vi "read_IMU_two_datasets_scaled.vi"(0 "First Measurement Type":u16(ring)=4608 items=["PAGE-ID"=0, "SYS_E_FLAG"=2048, "DIAG_STS"=2560, "ALM_STS"=3072, "TEMP_OUT"=3584, "X_GYRO_OUT"=4608, "Y_GYRO_OUT"=5632, "Z_GYRO_OUT"=6656, "X_ACCL_OUT"=7680, "Y_ACCL_OUT"=8704, "Z_ACCL_OUT"=9728, "X_MAGN_OUT"=10240, "Y_MAGN_OUT"=10752, "Z_MAGN_OUT"=11264, "BAROM_OUT"=12288, "X_DELTAANG_OUT"=16896, "Y_DELTAANG_OUT"=17920, "Z_DELTAANG_OUT"=18944, "X_DELTAVEL_OUT"=19968, "Y_DELTAVEL_OUT"=20992, "Z_DELTAVEL_OUT"=22016], 3 "Last Measurement Type":u16(ring)=4608 items=["PAGE-ID"=0, "SYS_E_FLAG"=2048, "DIAG_STS"=2560, "ALM_STS"=3072, "TEMP_OUT"=3584, "X_GYRO_OUT"=4608, "Y_GYRO_OUT"=5632, "Z_GYRO_OUT"=6656, "X_ACCL_OUT"=7680, "Y_ACCL_OUT"=8704, "Z_ACCL_OUT"=9728, "X_MAGN_OUT"=10240, "Y_MAGN_OUT"=10752, "Z_MAGN_OUT"=11264, "BAROM_OUT"=12288, "X_DELTAANG_OUT"=16896, "Y_DELTAANG_OUT"=17920, "Z_DELTAANG_OUT"=18944, "X_DELTAVEL_OUT"=19968, "Y_DELTAVEL_OUT"=20992, "Z_DELTAVEL_OUT"=22016], 7 "Gravitation-Constant":dbl=9.81, 9 "Next Measurement Type":u16(ring)=4608 items=["PAGE-ID"=0, "SYS_E_FLAG"=2048, "DIAG_STS"=2560, "ALM_STS"=3072, "TEMP_OUT"=3584, "X_GYRO_OUT"=4608, "Y_GYRO_OUT"=5632, "Z_GYRO_OUT"=6656, "X_ACCL_OUT"=7680, "Y_ACCL_OUT"=8704, "Z_ACCL_OUT"=9728, "X_MAGN_OUT"=10240, "Y_MAGN_OUT"=10752, "Z_MAGN_OUT"=11264, "BAROM_OUT"=12288, "X_DELTAANG_OUT"=16896, "Y_DELTAANG_OUT"=17920, "Z_DELTAANG_OUT"=18944, "X_DELTAVEL_OUT"=19968, "Y_DELTAVEL_OUT"=20992, "Z_DELTAVEL_OUT"=22016], 11 "error in (no error)":errorcluster) -> (1 "Sensor 1":string, 5 "Unit  1":string, 6 "Scaled Measurement 1":dbl, 10 "Scaled last Measurement":dbl, 12 "Last Sensor":string, 14 "error out":errorcluster, 15 "Last Unit":string)   [LabVIEW 2013]
panel:
  out "Error array 2":bool[](array[boolean])
  out "Error  array 1":bool[](array[boolean])
  out "1st Dataset":i16
  out "Last Dataset":i16
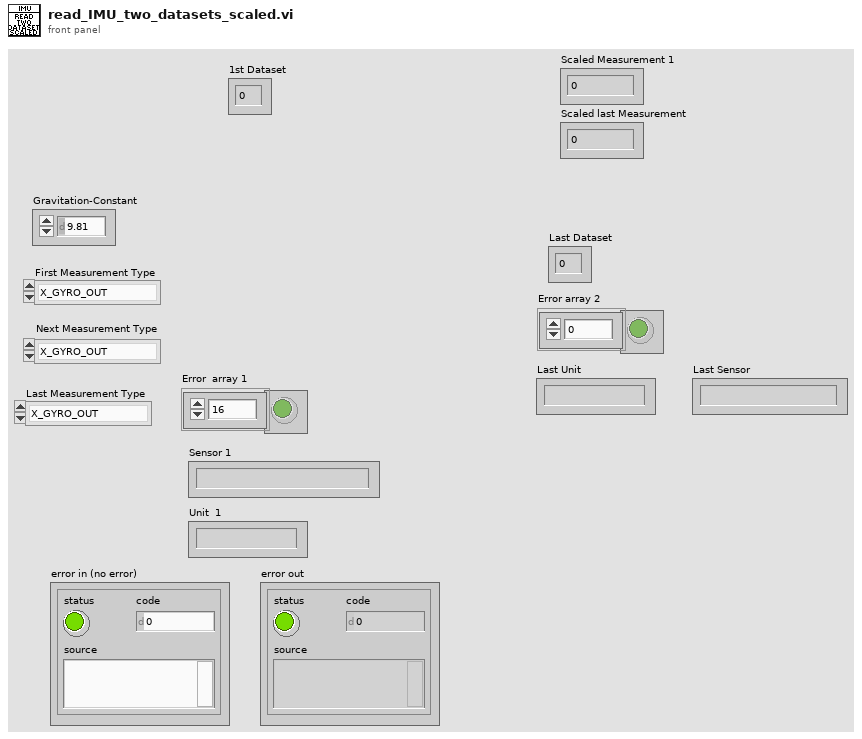
[diagram p1: front panel]
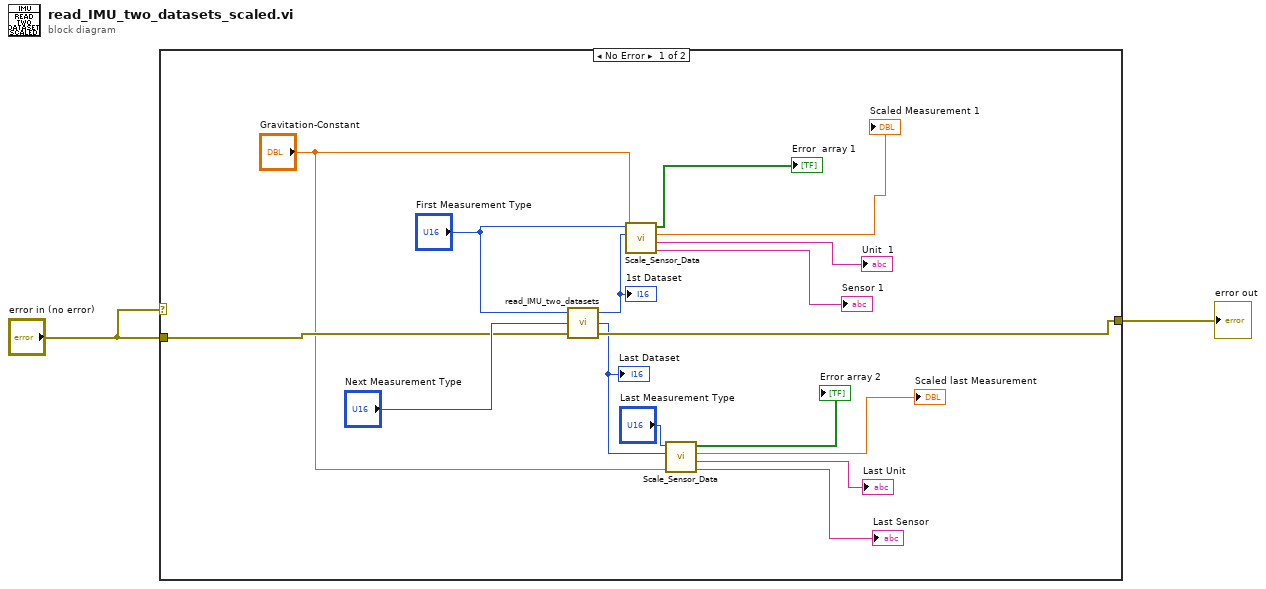
[diagram p0: block diagram]
diagram:
  n1 = case shown="No Error" "error in (no error)" {
    tunnel: [w18 w19] -> w2
    tunnel: "error in (no error)" -> [w9 w19]
    frame No Error {
      n2 = call "read_IMU_two_datasets.vi"("error in (no error)"=w9, "Next Measurement Type"="Next Measurement Type", "First Measurement Type"="First Measurement Type") -> ("error out"=w18:errorcluster, "Last Dataset"=w13:i16, "1st Dataset"=w10:i16)
      "Last Dataset" <- w13
      "1st Dataset" <- w10
      n3 = call "Scale_Sensor_Data.vi"("Gravitation-Constant"="Gravitation-Constant", "Dataset"=w10, "Measurement Type"="First Measurement Type") -> ("Sensor"=→"Sensor 1":string, "Unit"=→"Unit  1":string, "Scaled Measurement"=→"Scaled Measurement 1":dbl, "Alarm Array"=→"Error  array 1":bool[])  [unwired: 5 in]
      n4 = call "Scale_Sensor_Data.vi"("Gravitation-Constant"="Gravitation-Constant", "Dataset"=w13, "Measurement Type"="Last Measurement Type") -> ("Sensor"=→"Last Sensor":string, "Unit"=→"Last Unit":string, "Scaled Measurement"=→"Scaled last Measurement":dbl, "Alarm Array"=→"Error array 2":bool[])  [unwired: 5 in]
    }
    frame Error {
    }
  }
  "error out" <- w2
